vi "Untitled 2 (SubVI) 1.vi"(11 "all rows":ext[][](array[numeric])) -> (1 "Array 2":ext[](array[numeric]), 2 "Numeric":ext, 3 "Array":ext[](array[numeric]))   [LabVIEW 2013]
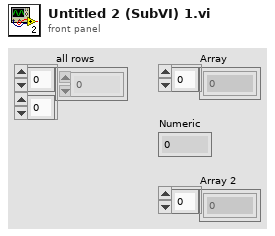
[diagram p1: front panel]
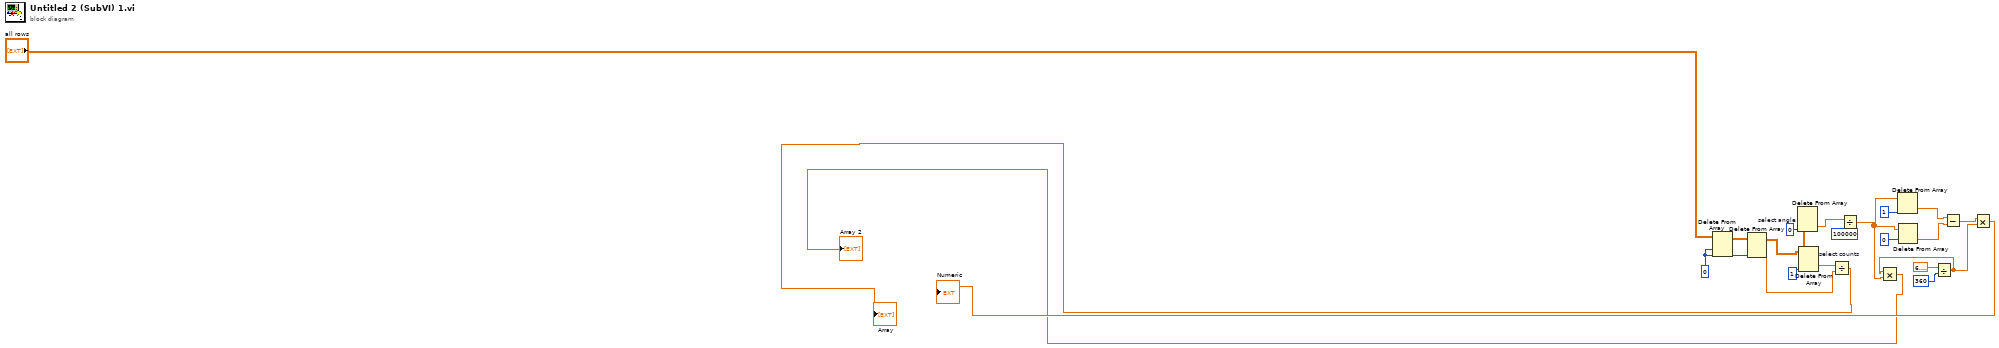
[diagram p0: block diagram]
diagram:
  w6 = 0
  n1 = Delete From Array(array="all rows", index (row)=w6) -> (array with subset deleted=w3:ext[][])  [unwired: 2 in, 1 out]
  n2 = Delete From Array(array=w3, index (col)=w6) -> (deleted portion=w7:ext[], array with subset deleted=w4:ext[][])  [unwired: 2 in]
  n3 = Delete From Array "select angle"(array=w4, index (col)=0) -> (deleted portion=w21:ext[])  [unwired: 2 in, 1 out]
  n4 = Delete From Array "select counts"(array=w4, index (col)=1) -> (deleted portion=w5:ext[])  [unwired: 2 in, 1 out]
  n5 = Divide(x=w5, y=w7) -> (x/y=→"Array":ext[])
  n6 = Divide(x=w21, y=100000) -> (x/y=w22:ext[])
  n7 = Delete From Array(array=w22, index=1) -> (deleted portion=w10:ext)  [unwired: 1 in, 1 out]
  n8 = Delete From Array(array=w22, index=0) -> (deleted portion=w11:ext)  [unwired: 1 in, 1 out]
  n9 = Divide(x=6.283185307179586, y=360) -> (x/y=w15:dbl)
  n10 = Multiply(x=w15, y=w22) -> (x*y=→"Array 2":ext[])
  n11 = Subtract(x=w10, y=w11) -> (x-y=w14:ext)
  n12 = Multiply(x=w14, y=w15) -> (x*y=→"Numeric":ext)
